vi "LVFunction_Get installed HASO sensor list.vi"(11 "error in (no error)":errorcluster) -> (4 "Array_Of_HASO_specifications":T5(array[cluster]), 6 "ArrayOfConfigFilePath":path[](array[path]), 8 "Installed sensors":string[](array[string]), 10 "HasoModelList":string[](array[string]))   [LabVIEW 2018]
uses:
  Controls/HasoSpecifications.ctl
  Controls/General dimensions definition.ctl
  Controls/Point2D.ctl
  Controls/Point2Df.ctl
  Tools/Remove Duplicates from 1D Array (String)__ogtk.vi
panel:
  in  "String 2":string
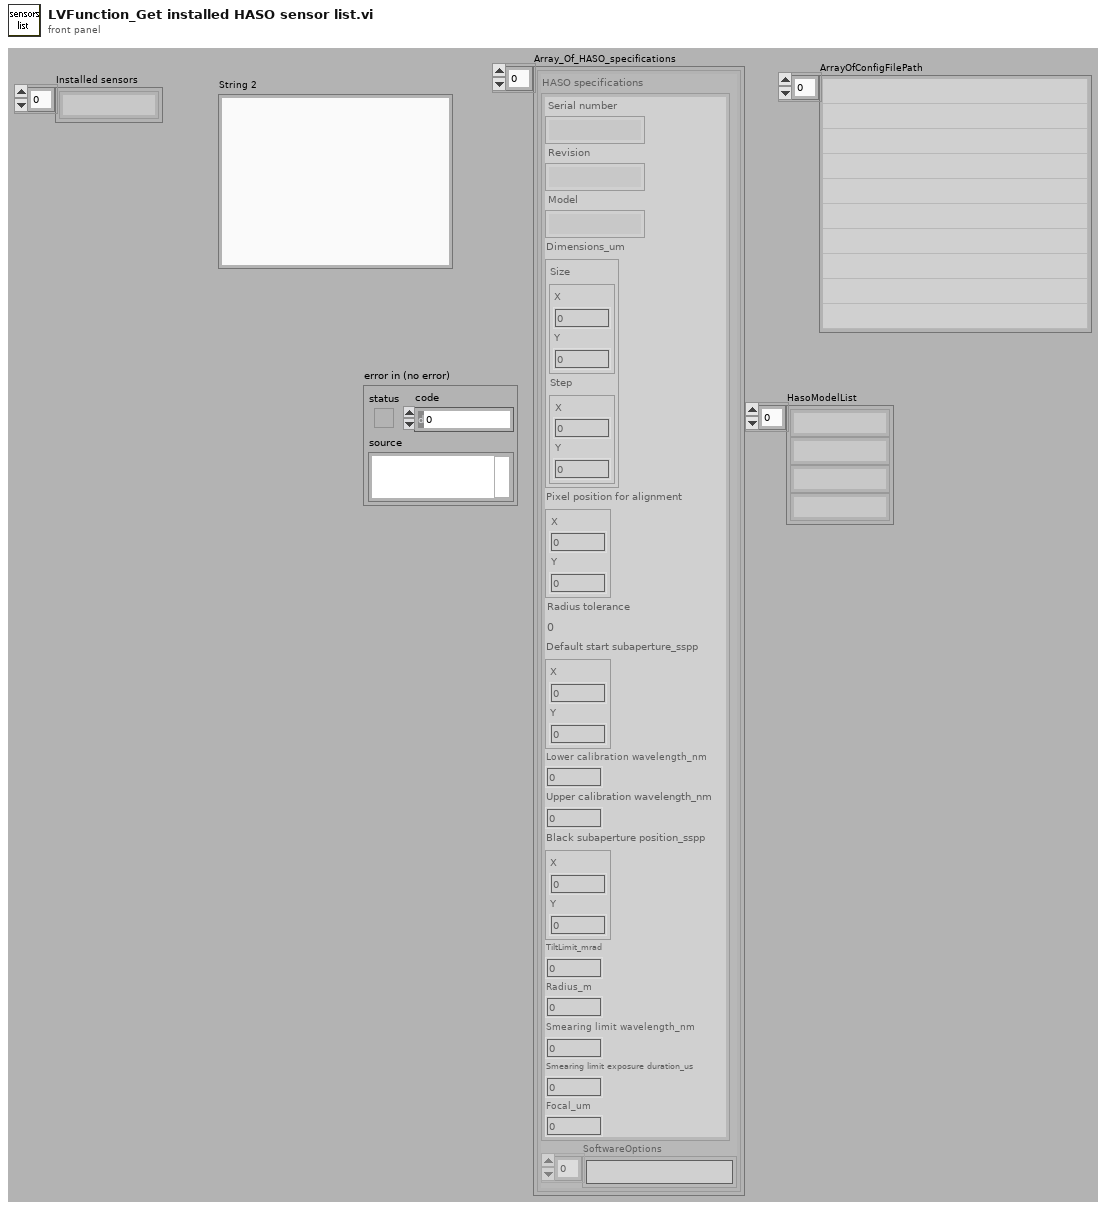
[diagram p1: front panel]
types:
  T1 = typedef "HasoSpecifications.ctl" = cluster{"Serial number":string, "Revision":string, "Model":string, "Dimensions_um":T2, "Pixel position for alignment":T4, "Radius tolerance":u16, "Default start subaperture_sspp":T3, "Lower calibration wavelength_nm":dbl, "Upper calibration wavelength_nm":dbl, "Black subaperture position_sspp":T3, "TiltLimit_mrad":dbl, "Radius_m":dbl, "Smearing limit wavelength_nm":dbl, "Smearing limit exposure duration_us":dbl, "Focal_um":dbl}
  T2 = typedef "General dimensions definition.ctl" = cluster{"Size":T3, "Step":T4}
  T3 = typedef "Point2D.ctl" = cluster{"X":u32, "Y":u32}
  T4 = typedef "Point2Df.ctl" = cluster{"X":sgl, "Y":sgl}
  T5 = cluster{"HASO specifications":T1, "SoftwareOptions":string[]}[]
  T6 = cluster{"HASO specifications":T1, "SoftwareOptionsList":string[]}
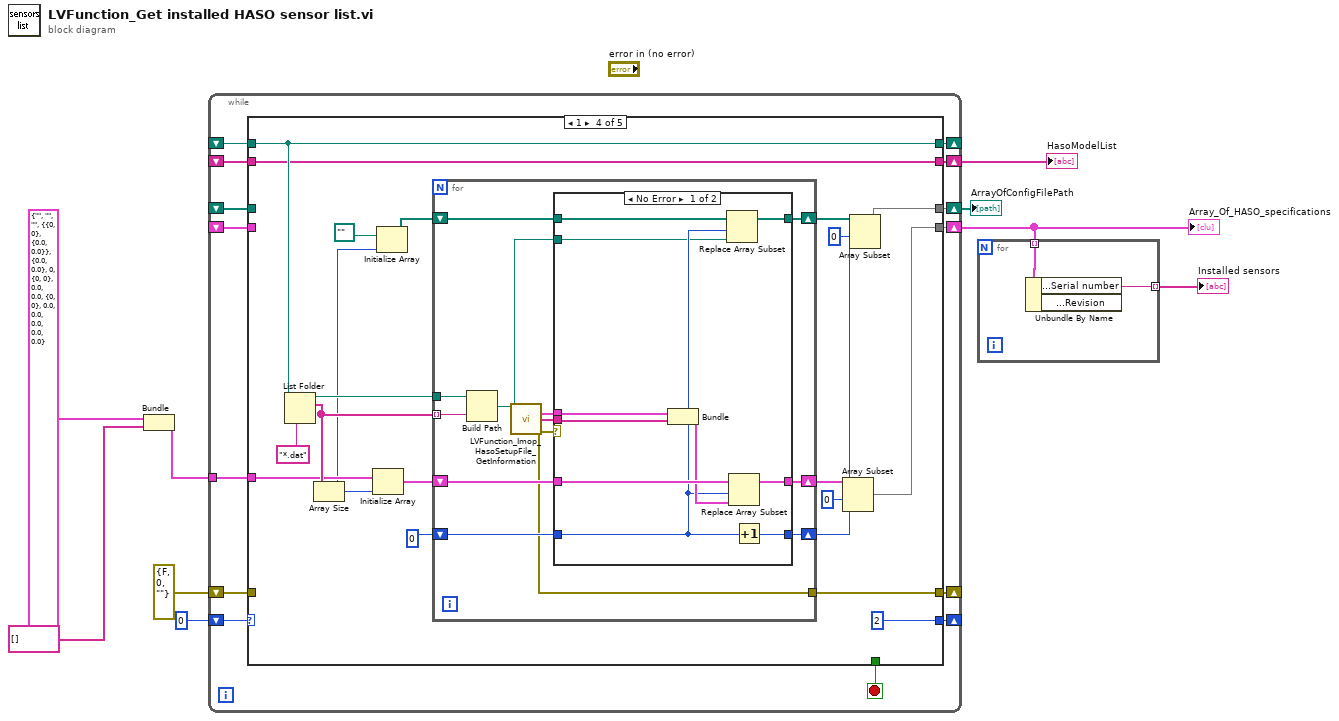
[diagram p0: block diagram]
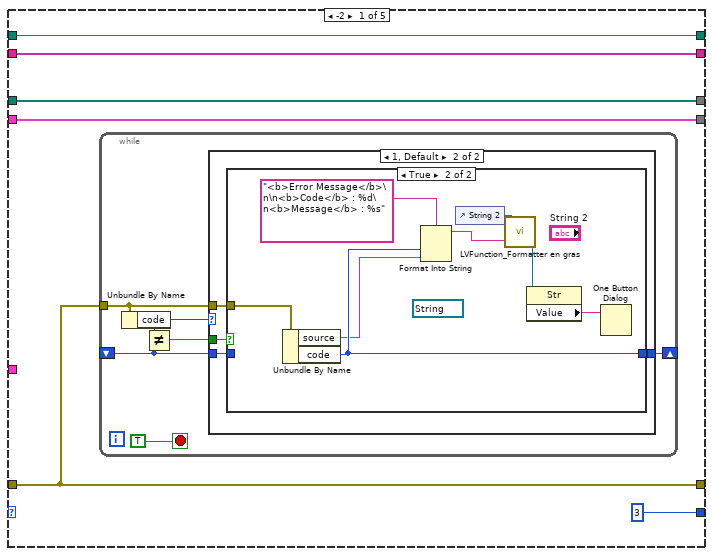
[diagram p2: hidden frame]
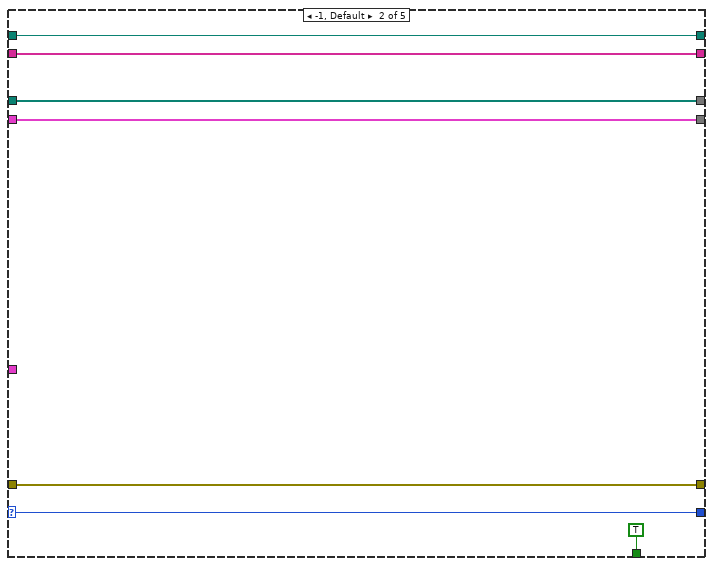
[diagram p5: hidden frame]
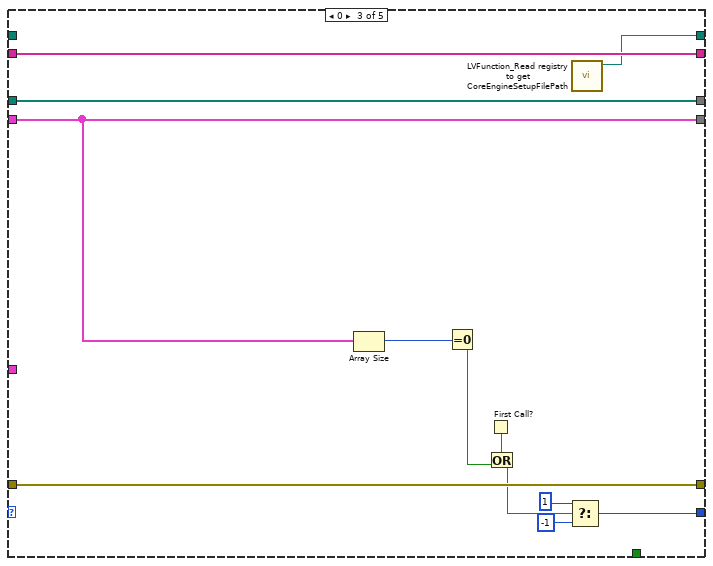
[diagram p6: hidden frame]
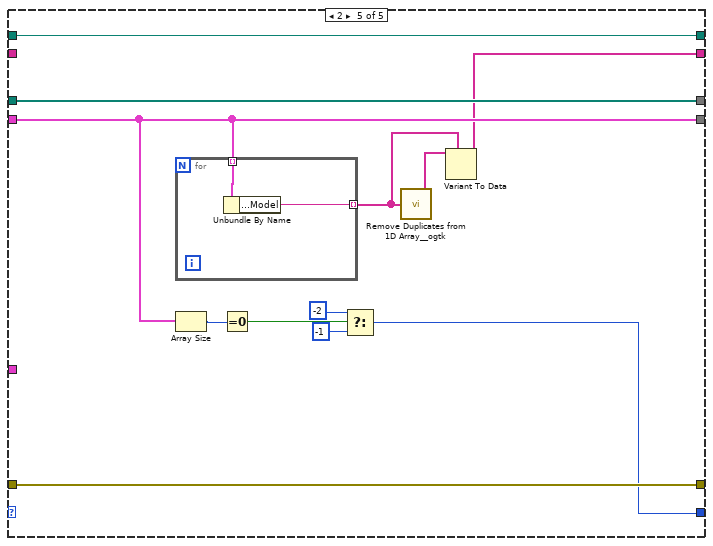
[diagram p8: hidden frame]
diagram:
  n1 = Bundle("HASO specifications"=T1 {"Serial number"="", "Revision"="", "Model"="", "Dimensions_um"={"Size"={"X"=0, "Y"=0}, "Step"={"X"=0.0, "Y"=0.0}}, "Pixel position for alignment"={"X"=0.0, "Y"=0.0}, "Radius tolerance"=0, "Default start subaperture_sspp"={"X"=0, "Y"=0}, "Lower calibration wavelength_nm"=0.0, "Upper calibration wavelength_nm"=0.0, "Black subaperture position_sspp"={"X"=0, "Y"=0}, "TiltLimit_mrad"=0.0, "Radius_m"=0.0, "Smearing limit wavelength_nm"=0.0, "Smearing limit exposure duration_us"=0.0, "Focal_um"=0.0}, string[] []) -> (w6:cluster{"HASO specifications":T1, string[]})  [unwired: 1 in]
  n2 = while {
    shift-right: [w18] -> _
    shift-left: 0 -> [w23]
    shift-right: [w21] -> w4
    shift-left: _ -> [w20]
    tunnel: w6 -> [w22]
    shift-right: [w16] -> _
    shift-left: errorcluster {"status"=FALSE, "code"=0, "source"=""} ("error out") -> [w17]
    shift-right: [w15] -> w2
    shift-left: _ -> [w14]
    shift-right: [w13] -> _
    shift-left: _ -> [w12]
    shift-right: [w11] -> w1
    shift-left: _ -> [w10]
    stop <- w19 stop-if-true
    n3 = case shown="1" w23 {
      selector: w23 -> [_ w54 _ _ _]
      tunnel: w22 -> [_ _ _ w85 _]
      tunnel: [w27 w56 w66 w81 w115] -> w21
      tunnel: w20 -> [w27 w56 w66 _ w115]
      tunnel: [_ TRUE _ _ _] -> w19
      tunnel: [3 w54 w62 2 w120] -> w18
      tunnel: w17 -> [w29 w53 w68 _ w125]
      tunnel: [w29 w53 w68 w78 w125] -> w16
      tunnel: [w26 w52 w67 w73 w124] -> w15
      tunnel: w14 -> [w26 w52 w67 _ w124]
      tunnel: [w25 w51 w57 w71 w123] -> w13
      tunnel: w12 -> [w25 w51 _ w71 w123]
      tunnel: [w24 w50 w58 w69 w114] -> w11
      tunnel: w10 -> [w24 w50 w58 w69 _]
      frame -2 {
        n4 = while {
          tunnel: w29 -> [w35]
          shift-right: [w34] -> _
          shift-left: _ -> [w33]
          stop <- TRUE stop-if-true
          n5 = Unbundle By Name(w35) -> ("code"=w30:i32)
          n6 = Not Equal?(x=w30, y=w33) -> (x != y?=w31:bool)
          n7 = case shown="1, Default" w30 {
            selector: w30 -> [w36 _]
            tunnel: w35 -> [_ w40]
            tunnel: [w36 w39] -> w34
            tunnel: w33 -> [_ w38]
            tunnel: w31 -> [_ w37]
            frame 0 {
            }
            frame 1, Default {
              n8 = case shown="True" w37 {
                tunnel: w40 -> [_ w49]
                tunnel: [w41 w48] -> w39
                tunnel: w38 -> [w41 _]
                frame False {
                }
                frame True {
                  (unwired) refnum<vi> refnum ("String to Format (not a refnum)")
                  n9 = Unbundle By Name(w49) -> ("source"=w47:string, "code"=w48:i32)
                  n10 = Format Into String(format string="<b>Error Message</b>\n\n<b>Code</b> : %d\n<b>Message</b> : %s" ("initial string"), w48, w47) -> (resulting string=w43:string)  [unwired: 2 in, 1 out]
                  n11 = control-ref of="String 2"() -> (w44:refnum<vi>)
                  n12 = call "LVFunction_Formatter en gras.vi"("Chaîne"=w43, "Contrôle chaîne"=w44) -> ("Contrôle chaîne (dup)"=w42:refnum<vi>)  [unwired: 1 in]
                  n13 = property class="Str"(reference=w42) -> ("Value"=w45:string)  [unwired: 1 in, 2 out]
                  n14 = One Button Dialog(message=w45) -> ()  [unwired: 1 in, 1 out]
                }
              }
            }
          }
        }
      }
      frame -1, Default {
      }
      frame 0 {
        n15 = Array Size(array=w66) -> (size(s)=w65:i32)
        n16 = Equal To 0?(x=w65) -> (x = 0?=w60:bool)
        n17 = First Call?() -> (First Call?: T/F=w61:bool)
        n18 = Or(x=w61, y=w60) -> (x .or. y?=w59:bool)
        n19 = Select(t=1, s=w59, f=-1) -> (s? t:f=w62:i32)
        n20 = call "LVFunction_Read registry to get CoreEngineSetupFilePath.vi"() -> ("Path to config files"=w57:path)  [unwired: 6 in, 1 out]
      }
      frame 1 {
        n21 = List Folder(path=w71, pattern="*.dat") -> (path out=w87:path, filenames=w86:string[])  [unwired: 2 in, 2 out]
        n22 = Array Size(array=w86) -> (size(s)=w77:i32)
        n23 = Initialize Array(w85, w77) -> (w84:cluster{"HASO specifications":T1, string[]}[])
        n24 = Initialize Array(path "" ("appended path"), w77) -> (w72:path[])
        n25 = for {
          tunnel: w87 -> [w100]
          tunnel: w86 -> [w99] mode=indexing
          shift-right: [w96] -> w82
          shift-left: w84 -> [w98]
          shift-right: [w93] -> w70
          shift-left: 0 -> [w97]
          tunnel: [w92] -> w78
          shift-right: [w90] -> w74
          shift-left: w72 -> [w91]
          n26 = Build Path(base path=w100, name or relative path=w99) -> (appended path=w89:path)
          n27 = call "LVFunction_Imop_HasoSetupFile_GetInformation.vi"("WFS_setup_file IN"=w89) -> ("HASO specifications"=w95:T1, "SoftwareOptionsList"=w94:string[], "error out"=w92:errorcluster)  [unwired: 10 in, 2 out]
          n28 = case shown="No Error" w92 {
            tunnel: w98 -> [w110 w113]
            tunnel: w97 -> [w104 w112]
            tunnel: [w109 w113] -> w96
            tunnel: w95 -> [w102 _]
            tunnel: w94 -> [w101 _]
            tunnel: [w107 w112] -> w93
            tunnel: w91 -> [w106 w111]
            tunnel: [w105 w111] -> w90
            tunnel: w89 -> [w103 _]
            frame No Error {
              n29 = Bundle("HASO specifications"=w102, "SoftwareOptionsList"=w101) -> (w108:T6)  [unwired: 1 in]
              n30 = Replace Array Subset(array=w106, new element=w103, index=w104) -> (w105:path[])
              n31 = Replace Array Subset(array=w110, new element=w108, index=w104) -> (w109:cluster{"HASO specifications":T1, string[]}[])
              n32 = Increment(x=w104) -> (x+1=w107:i32)
            }
            frame Error {
            }
          }
        }
        n33 = Array Subset(array=w82, index=0, length=w70) -> (w81:cluster{"HASO specifications":T1, string[]}[])
        n34 = Array Subset(array=w74, index=0, length=w70) -> (w73:path[])
      }
      frame 2 {
        n35 = for {
          tunnel: w115 -> [w127] mode=indexing
          tunnel: [w126] -> w116 mode=indexing
          n36 = Unbundle By Name(w127) -> ("HASO specifications.Model"=w126:string)
        }
        n37 = Array Size(array=w115) -> (size(s)=w122:i32)
        n38 = Equal To 0?(x=w122) -> (x = 0?=w121:bool)
        n39 = Select(t=-2, s=w121, f=-1) -> (s? t:f=w120:i32)
        n40 = call-poly "Remove Duplicates from 1D Array__ogtk.vi"("Input Array"=w116) -> ("Output Array"=w117:string[])  [unwired: 1 out]
        n41 = Variant To Data(type=w116, Variant=w117) -> (data=w114:string[])  [unwired: 1 in, 1 out]
      }
    }
  }
  "Array_Of_HASO_specifications" <- w4
  "ArrayOfConfigFilePath" <- w2
  "HasoModelList" <- w1
  n42 = for {
    tunnel: w4 -> [w129] mode=indexing
    tunnel: [w128] -> w3 mode=indexing
    n43 = Unbundle By Name(w129) -> ("HASO specifications.Serial number"=w128:string)  [unwired: 1 out]
  }
  "Installed sensors" <- w3
